vi "LoadController.vi"(8 "error in (no error)":errorcluster, 10 "Actor In":refnum<class "Actor.lvclass">, 11 "DemoStage in":refnum<class "DemoStage.lvclass">) -> (0 "error out":errorcluster, 3 "DemoStage out":refnum<class "DemoStage.lvclass">)   [LabVIEW 2020, in "DemoStage.lvlib" / "DemoStage.lvclass"]
uses:
  DemoStage.lvclass
  <vilib>/ActorFramework/Actor/Actor.lvclass
  ViewController/TripleAxisStageController/TripleAxisStageController.lvclass
  C:/Program Files/National Instruments/LabVIEW 2020/vi.lib/ActorFramework/Actor/Actor.lvclass
  Hardware Abstraction Layer/Component/Stage/Stage/Stage.lvclass
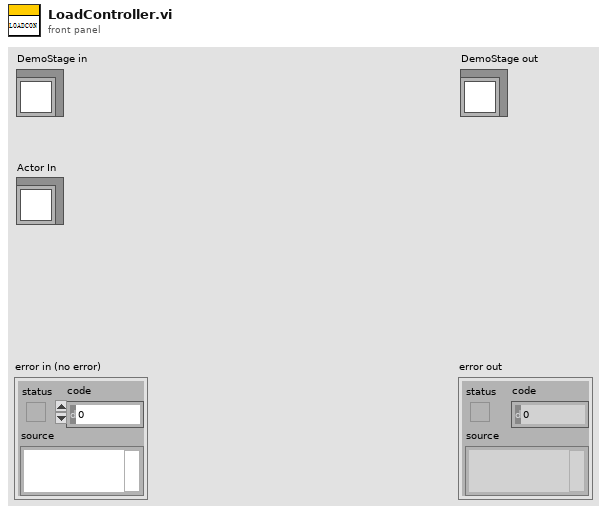
[diagram p1: front panel]
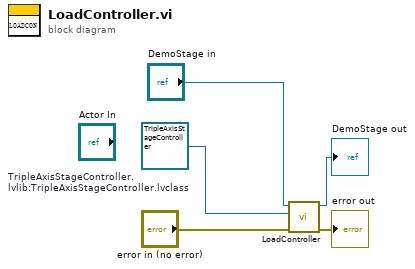
[diagram p0: block diagram]
diagram:
  w1 = refnum<class "TripleAxisStageController.lvclass"> refnum  # TripleAxisStageController.lvlib:TripleAxisStageController.lvclass
  n1 = call-parent "LoadController.vi"("error in (no error)"="error in (no error)", "Actor In"=w1, "Device in"="DemoStage in") -> ("error out"=→"error out":errorcluster, "Device out"=→"DemoStage out":refnum<class "DemoStage.lvclass">)  [unwired: 7 in]
